vi "hogeghoge.vi"() -> ()   [LabVIEW 2024]
panel:
  out "string":string
  out "Array 4":u32[](array[numeric]) format="%x"
  out "Array 3":string[](array[string])
  out "read buffer 4":string
  in  "read buffer 2":string
  out "Array 2":u32[](array[numeric]) format="%x"
  out "Array":string[](array[string])
  out "read buffer 3":string
  in  "read buffer":string
  out "Bcc":string
  out "GyroZ":string
  out "GyroY":string
  out "GyroX":string
  out "AccZ":string
  out "AccY":string
  out "AccX":string
  out "ticktime":string
  out "comand":string
  out "Head":string
  in  "stop":bool
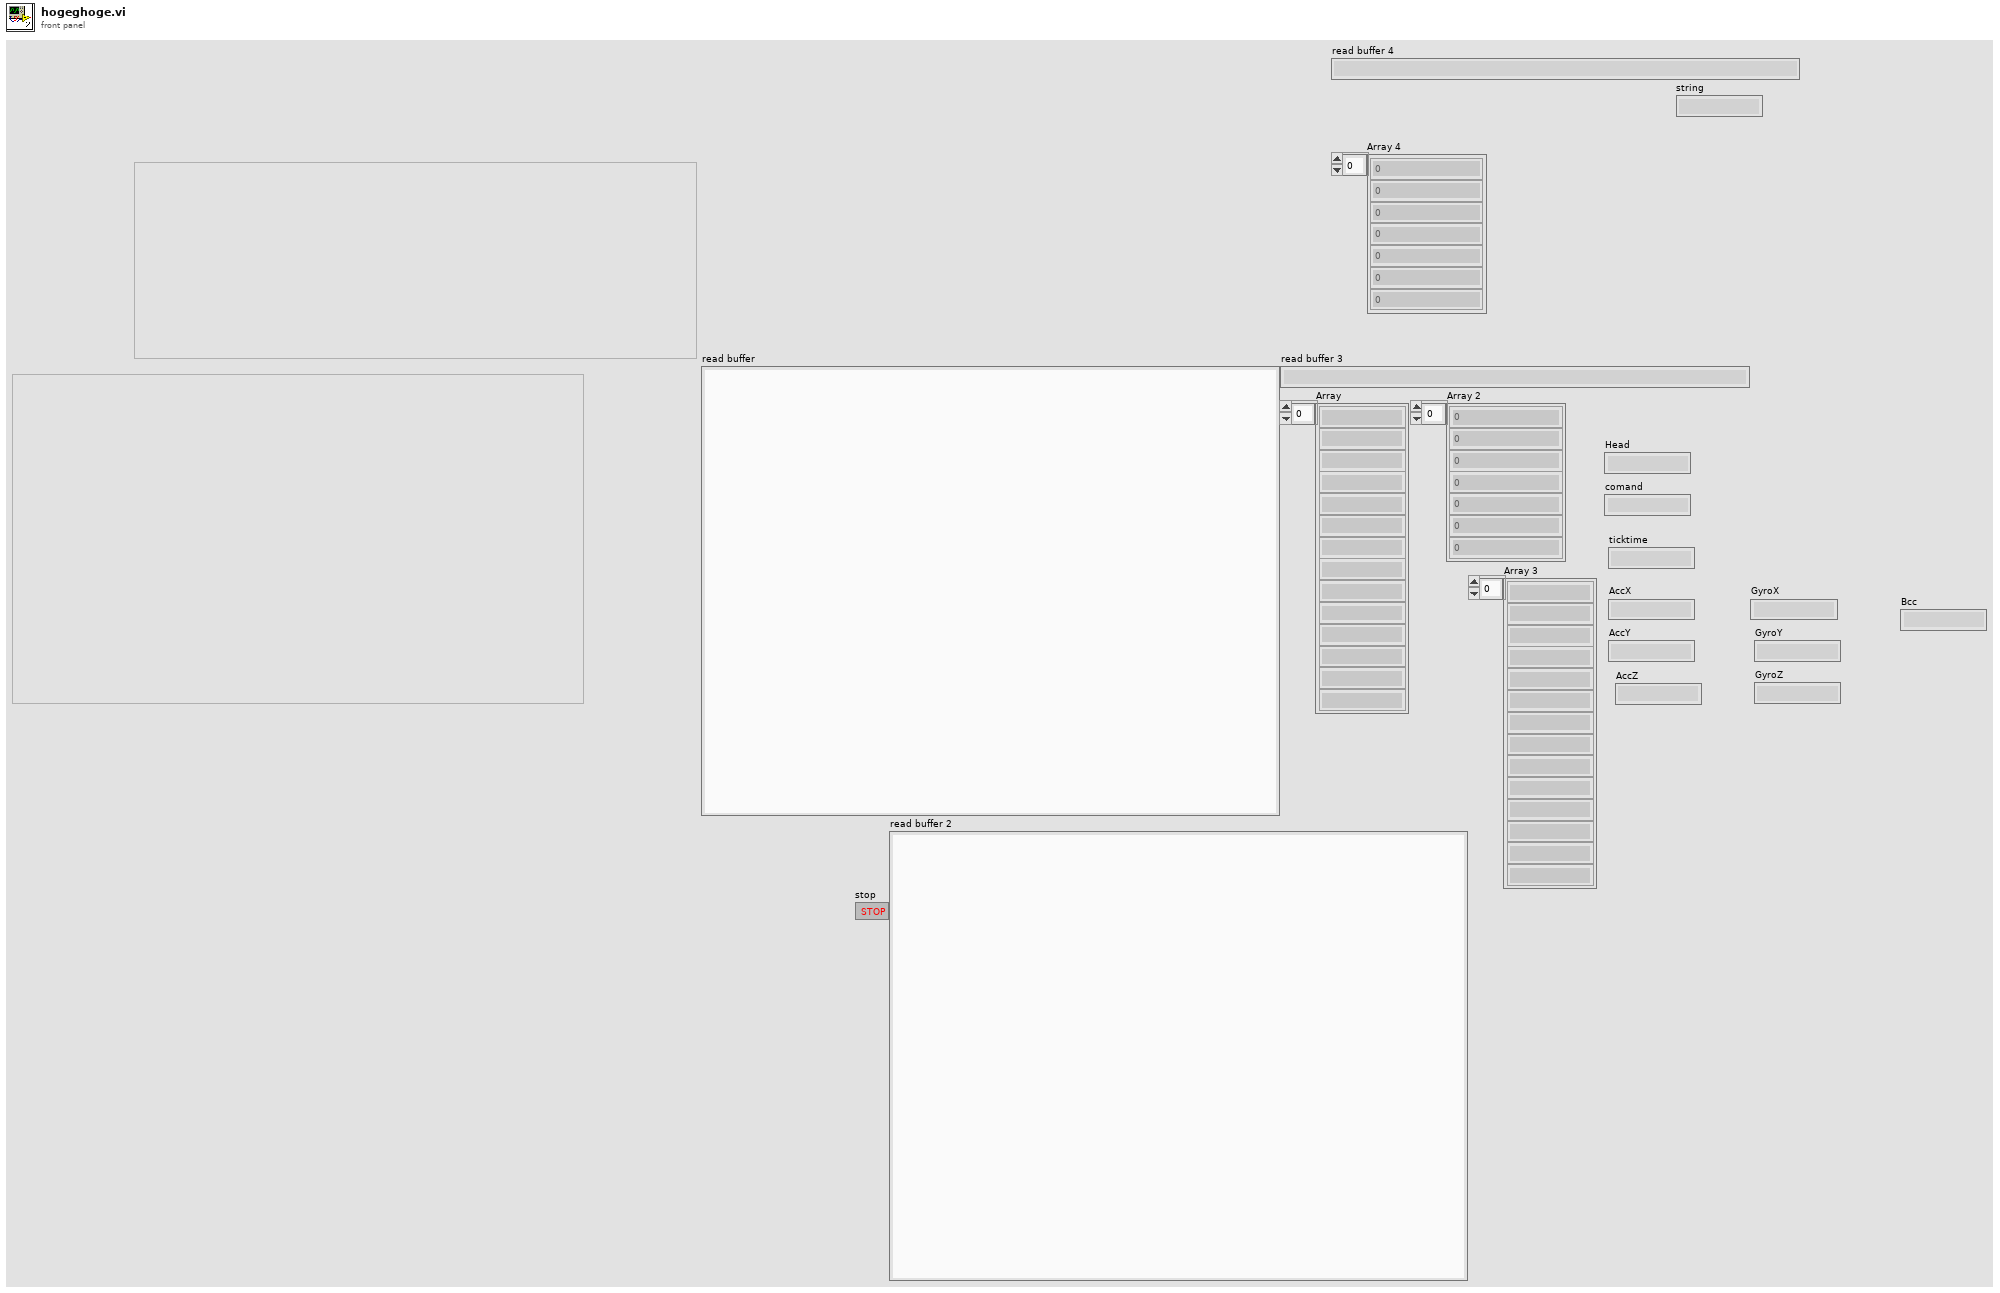
[diagram p1: front panel]
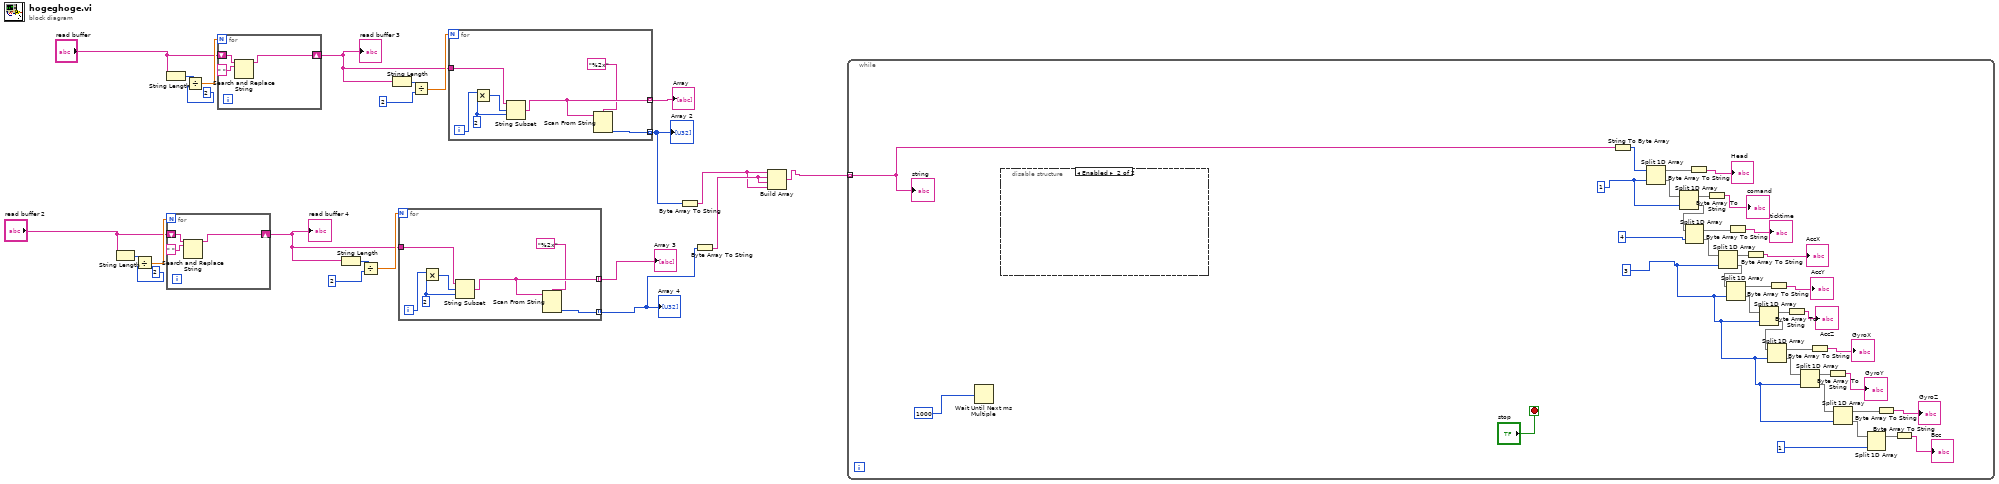
[diagram p0: block diagram]
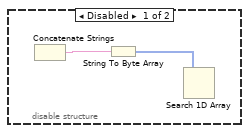
[diagram p2: hidden frame]
diagram:
  n1 = String Length(string="read buffer 2") -> (length=w13:i32)
  n2 = Divide(x=w13, y=2) -> (x/y=w11:dbl)
  n3 = String Length(string="read buffer") -> (length=w23:i32)
  n4 = for {
    N: w11 -> [_]
    shift-right: [w24] -> w6
    shift-left: "read buffer 2" -> [w25]
    n5 = Search and Replace String(input string=w25, search string=" ") -> (result string=w24:string)  [unwired: 6 in, 3 out]
  }
  "read buffer 4" <- w6
  n6 = Divide(x=w23, y=2) -> (x/y=w21:dbl)
  n7 = for {
    N: w21 -> [_]
    shift-right: [w27] -> w16
    shift-left: "read buffer" -> [w28]
    n8 = Search and Replace String(input string=w28, search string=" ") -> (result string=w27:string)  [unwired: 6 in, 3 out]
  }
  "read buffer 3" <- w16
  n9 = String Length(string=w6) -> (length=w9:i32)
  n10 = Divide(x=w9, y=2) -> (x/y=w7:dbl)
  n11 = String Length(string=w16) -> (length=w19:i32)
  n12 = for {
    N: w7 -> [_]
    tunnel: w6 -> [w33]
    tunnel: [w32] -> w5 mode=indexing
    tunnel: [w30] -> w4 mode=indexing
    i -> [w35]
    w34 = 2
    n13 = Multiply(x=w35, y=w34) -> (x*y=w36:i32)
    n14 = String Subset(string=w33, offset (0)=w36, length (rest)=w34) -> (substring=w32:string)
    n15 = Scan From String(format string="%2x", input string=w32) -> (output 1=w30:u32)  [unwired: 3 in, 3 out]
  }
  "Array 3" <- w5
  "Array 4" <- w4
  n16 = Divide(x=w19, y=2) -> (x/y=w17:dbl)
  n17 = for {
    N: w17 -> [_]
    tunnel: w16 -> [w40]
    tunnel: [w39] -> w15 mode=indexing
    tunnel: [w37] -> w14 mode=indexing
    i -> [w42]
    w41 = 2
    n18 = Multiply(x=w42, y=w41) -> (x*y=w43:i32)
    n19 = String Subset(string=w40, offset (0)=w43, length (rest)=w41) -> (substring=w39:string)
    n20 = Scan From String(format string="%2x", input string=w39) -> (output 1=w37:u32)  [unwired: 3 in, 3 out]
  }
  "Array" <- w15
  "Array 2" <- w14
  n21 = Byte Array To String(unsigned byte array=w14) -> (string=w1:string)
  n22 = Byte Array To String(unsigned byte array=w4) -> (string=w2:string)
  n23 = Build Array(w1, w2, w2, w1) -> (w3:string[])
  n24 = while {
    tunnel: w3 -> [w44] mode=indexing
    stop <- "stop" stop-if-true
    w47 = 3
    w74 = 1
    n25 = Wait Until Next ms Multiple(millisecond multiple=u32 1000) -> ()  [unwired: 1 out]
    n26 = disable-structure shown="Enabled" {
      frame Disabled {
        n27 = Concatenate Strings() -> (w81:string, w84:string, w83:string)
        n28 = String To Byte Array(string=w81) -> (unsigned byte array=w82:u8[])
        n29 = Search 1D Array(1D array=w82) -> ()  [unwired: 2 in, 1 out]
      }
      frame Enabled {
      }
    }
    n30 = String To Byte Array(string=w44) -> (unsigned byte array=w78:u8[])
    n31 = Split 1D Array(array=w78, index=w74) -> (first subarray=w77:u8[], second subarray=w75:u8[])
    n32 = Split 1D Array(array=w75, index=w74) -> (first subarray=w73:u8[], second subarray=w56:u8[])
    n33 = Split 1D Array(array=w56, index=4) -> (first subarray=w71:u8[], second subarray=w69:u8[])
    n34 = Byte Array To String(unsigned byte array=w77) -> (string=→"Head":string)
    n35 = Byte Array To String(unsigned byte array=w73) -> (string=→"comand":string)
    n36 = Split 1D Array(array=w69, index=w47) -> (first subarray=w68:u8[], second subarray=w55:u8[])
    n37 = Split 1D Array(array=w55, index=w47) -> (first subarray=w66:u8[], second subarray=w64:u8[])
    n38 = Byte Array To String(unsigned byte array=w71) -> (string=→"ticktime":string)
    n39 = Byte Array To String(unsigned byte array=w68) -> (string=→"AccX":string)
    n40 = Split 1D Array(array=w64, index=w47) -> (first subarray=w63:u8[], second subarray=w54:u8[])
    n41 = Split 1D Array(array=w54, index=w47) -> (first subarray=w61:u8[], second subarray=w59:u8[])
    n42 = Byte Array To String(unsigned byte array=w66) -> (string=→"AccY":string)
    n43 = Byte Array To String(unsigned byte array=w63) -> (string=→"AccZ":string)
    n44 = Split 1D Array(array=w59, index=w47) -> (first subarray=w58:u8[], second subarray=w48:u8[])
    n45 = Byte Array To String(unsigned byte array=w61) -> (string=→"GyroX":string)
    n46 = Byte Array To String(unsigned byte array=w58) -> (string=→"GyroY":string)
    n47 = Split 1D Array(array=w48, index=w47) -> (first subarray=w53:u8[], second subarray=w51:u8[])
    n48 = Split 1D Array(array=w51, index=1) -> (first subarray=w50:u8[])  [unwired: 1 out]
    n49 = Byte Array To String(unsigned byte array=w53) -> (string=→"GyroZ":string)
    n50 = Byte Array To String(unsigned byte array=w50) -> (string=→"Bcc":string)
    "string" <- w44
  }
